vi "Sum Last 5.vi"(10 "Input":dbl) -> (3 "Sum Last 5":dbl)   [LabVIEW 2012]
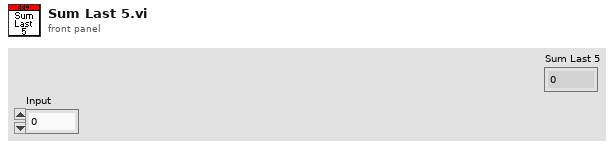
[diagram p1: front panel]
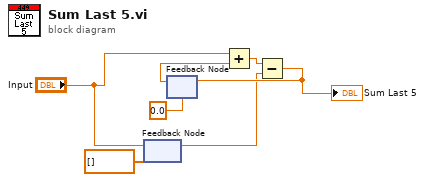
[diagram p0: block diagram]
diagram:
  n1 = feedback #1(dbl[] []) -> (w2:dbl)
  n2 = feedback-in #1("Input") -> ()
  n3 = feedback #2(0.0 ("max queue size (-1, unlimited)")) -> (w6:dbl)
  n4 = Add(x="Input", y=w6) -> (x+y=w5:dbl)
  n5 = Subtract(x=w5, y=w2) -> (x-y=w4:dbl)
  "Sum Last 5" <- w4
  n6 = feedback-in #2(w4) -> ()
